vi "QCP_TuningModeSet.vi"(8 "error in (no error)":errorcluster, 10 "On?":bool, 11 "QCP_DevRef_In":T1) -> (0 "error out":errorcluster, 3 "QCP_DevRef_Out":T1)   [LabVIEW 2016]
uses:
  <userlib>/836-libraries/System/QCP_V2/QCPSupportCode/QCP_RefNum.ctl
  <userlib>/836-libraries/System/QCP_V2/QCPSupportCode/QCPData.ctl
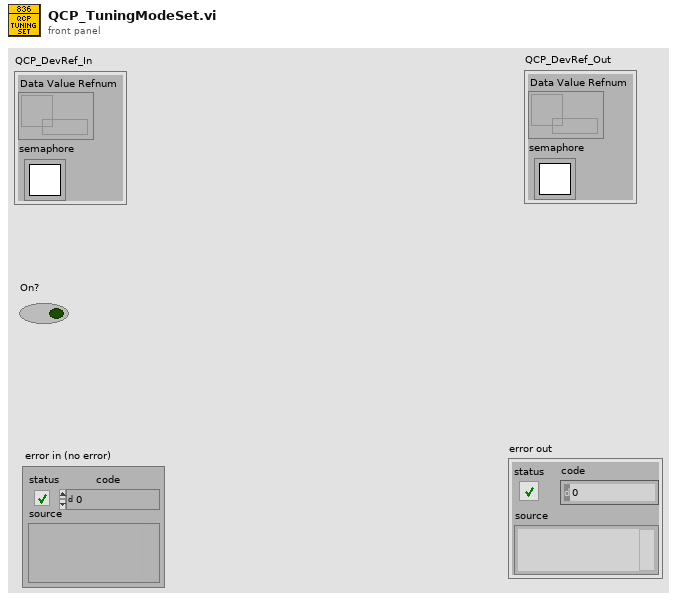
[diagram p1: front panel]
types:
  T1 = typedef "QCP_RefNum.ctl" = cluster{"Data Value Refnum":refnum<data-value>, "semaphore":T2}
  T2 = typedef "Semaphore RefNum" = refnum<k1>
  T3 = typedef "QCPData.ctl" = cluster{"Names":string[], "Values":cluster{"Array":dbl[]}[], "TuningMode?":bool}
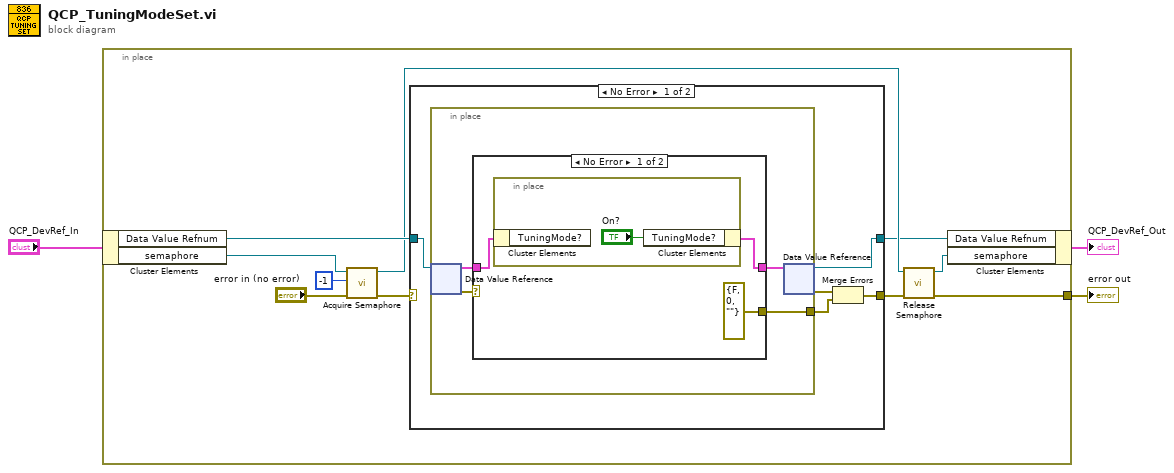
[diagram p0: block diagram]
diagram:
  n1 = in-place {
    in-place-border: [w5] -> w2
    n2 = in-place-cluster #1("QCP_DevRef_In") -> ("Data Value Refnum"=w9:refnum<data-value>, "semaphore"=w13:T2)
    n3 = call <vilib>:"Acquire Semaphore.vi"("error in (no error)"="error in (no error)", "ms timeout (-1)"=-1, "semaphore"=w13) -> ("error out"=w10:errorcluster, "semaphore out"=w7:T2)  [unwired: 2 in, 1 out]
    n4 = case shown="No Error" w10 {
      selector: w10 -> [_ w30]
      tunnel: w9 -> [w18 w29]
      tunnel: [w14 w30] -> w8
      tunnel: [w17 w29] -> w4
      frame No Error {
        n5 = in-place {
          in-place-border: [w19] -> w15
          n6 = in-place-dvr #2(w18) -> (w21:T3, w22:errorcluster)
          n7 = case shown="No Error" w22 {
            selector: w22 -> [_ w27]
            tunnel: w21 -> [w25 w28]
            tunnel: [w24 w28] -> w20
            tunnel: [errorcluster {"status"=FALSE, "code"=0, "source"=""} ("error IO") w27] -> w19
            frame No Error {
              n8 = in-place {
                n9 = in-place-cluster #3(w25) -> ()  [unwired: 1 out]
                n10 = in-place-cluster #3("TuningMode?"="On?") -> (w24:T3)
              }
            }
            frame Error {
            }
          }
          n11 = in-place-dvr #2(w20) -> (w17:refnum<data-value>, w16:errorcluster)
        }
        n12 = Merge Errors(w16, w15) -> (w14:errorcluster)
      }
      frame Error {
      }
    }
    n13 = call <vilib>:"Release Semaphore.vi"("error in (no error)"=w8, "semaphore"=w7) -> ("error out"=w5:errorcluster, "semaphore out"=w6:T2)  [unwired: 4 in]
    n14 = in-place-cluster #1("Data Value Refnum"=w4, "semaphore"=w6) -> (→"QCP_DevRef_Out":T1)
  }
  "error out" <- w2
